vi "Test Queue-Event.vi"() -> ()   [LabVIEW 2021]
panel:
  in  "add case":dbl
  in  "Numeric":i32
  out "Timeout number":u32
  out "Passed number":u32
  in  "Queued number":u32
  in  "ok to queue":bool
  in  "stop 2":bool
  in  "stop":bool
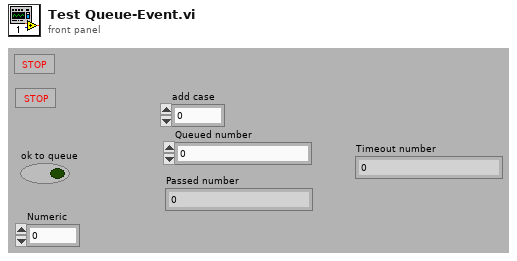
[diagram p1: front panel]
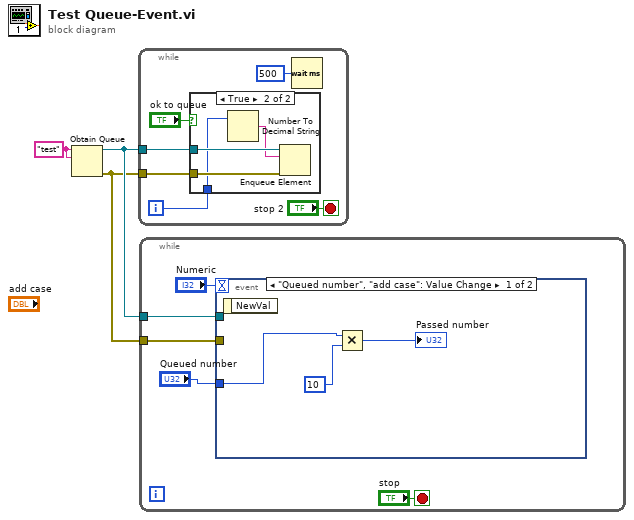
[diagram p0: block diagram]
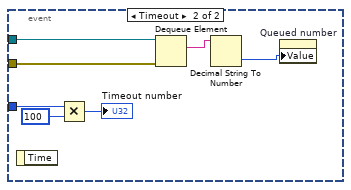
[diagram p3: hidden frame]
diagram:
  w3 = "test" ("name (unnamed)")
  n1 = Obtain Queue(name (unnamed)=w3, element data type=w3) -> (queue out=w2:refnum<queue>, error out=w1:errorcluster)  [unwired: 3 in, 1 out]
  n2 = while {
    tunnel: w2 -> [w8]
    tunnel: w1 -> [w7]
    i -> [w4]
    stop <- "stop 2" stop-if-true
    n3 = case shown="True" "ok to queue" {
      tunnel: w8 -> [_ w13]
      tunnel: w7 -> [_ w12]
      tunnel: w4 -> [_ w11]
      frame False {
      }
      frame True {
        n4 = Number To Decimal String(number=w11) -> (decimal integer string=w10:string)  [unwired: 1 in]
        n5 = Enqueue Element(queue=w13, element=w10, error in (no error)=w12) -> ()  [unwired: 1 in, 3 out]
      }
    }
    n6 = Wait (ms)(milliseconds to wait=u32 500) -> ()  [unwired: 1 out]
  }
  n7 = while {
    tunnel: w2 -> [w16]
    tunnel: w1 -> [w15]
    stop <- "stop" stop-if-true
    n8 = event shown="[0] \"Queued number\", \"add case\": Value Change" {
      selector: _ -> [_ _]
      dyn-events: _ -> [_ _]
      timeout: "Numeric" -> [_ _]
      tunnel: "Queued number" -> [w19 w27]
      tunnel: w16 -> [_ w23]
      tunnel: w15 -> [_ w22]
      event "Queued number", "add case": Value Change {
        n9 = event-data() -> ()  [unwired: 1 in, 1 out]
        n10 = Multiply(x=w19, y=u32 10) -> (x*y=→"Passed number":u32)
      }
      event Timeout {
        n11 = event-data() -> ()  [unwired: 1 in, 1 out]
        n12 = Multiply(x=w27, y=u32 100) -> (x*y=→"Timeout number":u32)
        n13 = Dequeue Element(queue=w23, error in (no error)=w22) -> (element=w24:string)  [unwired: 1 in, 3 out]
        n14 = Decimal String To Number(string=w24) -> (number=w25:i32)  [unwired: 2 in, 1 out]
        n15 = property on="Queued number" class="DigNum (strict)"("Value"=w25) -> ()  [unwired: 2 in, 2 out]
      }
    }
  }
